vi "Update Message Routing Info.vi"(0 "message":T1, 5 "receiver host (\"\")":string, 7 "receiver process (\"\")":string, 11 "error in":errorcluster, 12 "source host (\"\")":string, 13 "source process (\"\")":string) -> (4 "message":T1, 15 "error out":errorcluster)   [LabVIEW 2013, in "AMC.lvlib"]
doc: "Specifies the routing information for an AMC message."
uses:
  AMC.lvlib
  Message.ctl
  <vilib>/NI/Tools/Keyed Array/KeyedArray.ctl
  <vilib>/NI/Tools/Keyed Array/Tools_KeyedArray.lvlib
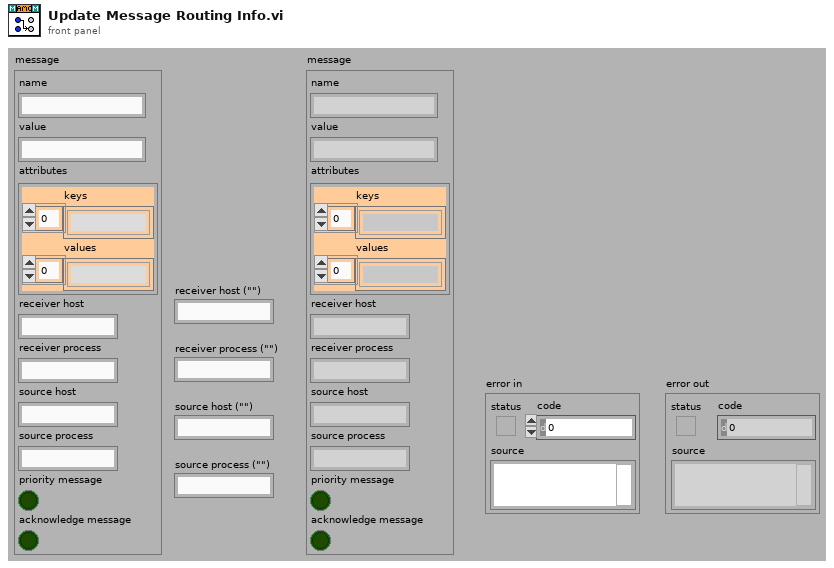
[diagram p1: front panel]
types:
  T1 = typedef "AMC.lvlib/Message.ctl" = cluster{"name":string, "value":string, "attributes":T2, "receiver host":string, "receiver process":string, "source host":string, "source process":string, "priority message":bool, "acknowledge message":bool}
  T2 = typedef "Tools_KeyedArray.lvlib/KeyedArray.ctl" = cluster{"keys":string[], "values":string[]}
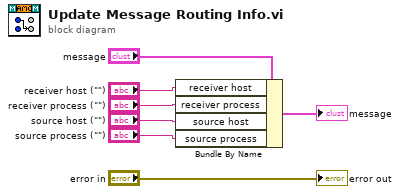
[diagram p0: block diagram]
diagram:
  n1 = Bundle By Name(cluster="message", "receiver host"="receiver host (\"\")", "receiver process"="receiver process (\"\")", "source host"="source host (\"\")", "source process"="source process (\"\")") -> (→"message":T1)
  "error out" <- "error in"
